vi "NI VeriStand - Parse Incoming Command Data.vi"(8 "error in (no error)":errorcluster, 11 "Incoming data":string) -> (0 "error out":errorcluster, 2 "Outgoing data":variant, 3 "Action":T1)   [LabVIEW 2020, in "Custom Device API.lvlib"]
doc: "Parses a <B>System Explorer</B> window user event and returns the appropriate <B>Action</B> command. You can wire the <B>Action</B> output to a Case Structure to configure how to respond to each command."
uses:
  <vilib>/NI VeriStand/Custom Device API/Custom Device API.lvlib
  <vilib>/NI VeriStand/Custom Device API/Custom Device Commands.ctl
  f9c8f758-b981-46c2-8b76-19f6e725d20a.vi
  <vilib>/NI VeriStand/Custom Device API/Custom Device Offline Path.vi
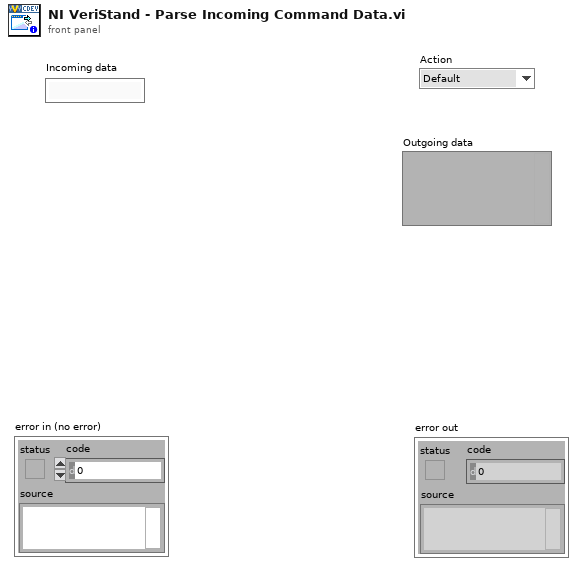
[diagram p1: front panel]
types:
  T1 = typedef "Custom Device API.lvlib/Custom Device Commands.ctl" = enum16{"Default", "Item renamed", "Shutdown", "Dynamic button pressed"}
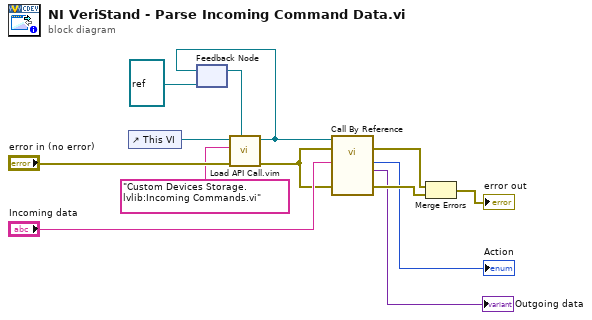
[diagram p0: block diagram]
diagram:
  n1 = control-ref of="This VI"() -> (w7:refnum<vi>)
  n2 = feedback #1(refnum<vi> refnum ("type specifier VI Refnum (for type only)")) -> (w8:refnum<vi>)
  n3 = call "Load API Call.vim"("VI reference in"=w8, "error in (no error)"="error in (no error)", "VI qualified name"="Custom Devices Storage.lvlib:Incoming Commands.vi", "Caller VI ref"=w7) -> ("error out"=w5:errorcluster, "VI reference"=w4:refnum<vi>)  [unwired: 6 in]
  n4 = feedback-in #1(w4) -> ()
  n5 = call-by-ref "?"(reference=w4, error in=w5, 8:"error in (no error)"=w5, "Data"="Incoming data") -> (error out=w1:errorcluster, 0:"error out"=w13:errorcluster, "Data"=→"Outgoing data":variant, "Action"=→"Action":T1)  [unwired: 7 in, 1 out]
  n6 = Merge Errors(w1, w13) -> (→"error out":errorcluster)
